vi "HFRR ADV v02.vi"() -> ()   [LabVIEW 2025] (continued)
            frame 9 {
            }
            frame 10 {
              n1911 = local write "Language Selection"(w2311) -> ()
            }
            frame 11 {
            }
            frame 12 {
            }
            frame 13 {
            }
            frame 14 {
            }
            frame 15 {
            }
            frame 16 {
            }
            frame 17 {
            }
            frame 18 {
            }
            frame 21 {
            }
            frame 22 {
              n1912 = local write "Com Port 3"(w2312) -> ()
            }
            frame 20 {
              n1913 = local write "Camera Port :"(w2313) -> ()
            }
            frame 19 {
              n1914 = local write "C3 :"(w2314) -> ()
            }
            frame 23, Default {
            }
          }
        }
      }
    }
    n1915 = Select(t=u32 2500 ("milliseconds to wait"), s=w2281, f=u32 500 ("milliseconds to wait")) -> (s? t:f=w2279:u32)
    n1916 = Multiply(x=w2284, y=w2279) -> (x*y=w2286:dbl)
    n1917 = call "Elapsed Time2"("Time Target (s)"=w2286, "Auto Reset"=TRUE) -> ("Time has Elapsed"=w2276:bool)  [unwired: 10 in, 7 out]
    n1918 = case shown="True" w2276 {
      frame False {
      }
      frame True {
        n1919 = stacked-sequence {
          frame #0 {
            # "DATA PROCESSING"
            # "115 mV/N"
            n1920 = local read "Sample Temperature 2"() -> (w2318:dbl)
            n1921 = local read "DEMO MODE"() -> (w2315:bool)
            n1922 = local read "RH Numeric:"() -> (→"Humidity ( %RH )":dbl)
            n1923 = local read "FRICVALZ"() -> (w2334:dbl)
            n1924 = local read "Friction"() -> (w2320:dbl)
            n1925 = call <vilib>:"Mean PtByPt.vi"("x"=w2318, "sample length"=100) -> ("mean"=w2317:dbl)  [unwired: 2 in, 1 out]
            "TEMP 2" <- w2317
            "TEMP 3" <- w2317
            n1926 = Subtract(x=w2320, y=w2334) -> (x-y=w2329:dbl)
            "FF 2" <- w2329
            "FF 4" <- w2329
            n1927 = case shown="False" w2315 {
              frame False {
                n1928 = local read "Ambient Temperature"() -> (→"AIR TEMP":dbl)
              }
              frame True {
              }
            }
            n1929 = local read "TEMP"() -> (w2333:dbl)
            n1930 = local write "FF 3"(w2329) -> ()
            n1931 = Compound Arithmetic op=OR("FRICVALZ 4", "FRICVALZ 3", "FRICVALZ 2") -> (w2325:bool)
            n1932 = case shown="True" w2325 {
              tunnel: w2320 -> [_ w2341]
              frame False {
              }
              frame True {
                w2340 = FALSE ("FRICVALZ")
                n1933 = local write "FRICVALZ 3"(w2340) -> ()
                n1934 = local write "FRICVALZ 2"(w2340) -> ()
                n1935 = local write "FRICVALZ 4"(w2340) -> ()
                "FRICVALZ" <- w2341
              }
            }
            n1936 = Not A Number/Path/Refnum?(number/path/refnum=w2333) -> (NaN/Path/Refnum?=w2332:bool)
            n1937 = Not A Number/Path/Refnum?(number/path/refnum=w2329) -> (NaN/Path/Refnum?=w2331:bool)
            n1938 = Divide(x=w2329, y=1.96) -> (x/y=w2326:dbl)
            n1939 = Compound Arithmetic op=OR(w2332, w2331) -> (w2330:bool)
            n1940 = Not A Number/Path/Refnum?(number/path/refnum=w2326) -> (NaN/Path/Refnum?=w2327:bool)
            n1941 = case shown="True" w2330 {
              frame False {
              }
              frame True {
                n1942 = local write "TEMP"(0.0 ("TEMP")) -> ()
                n1943 = local write "FF 2"(0.0 ("FF 2")) -> ()
                n1944 = local write "reinit"(TRUE ("reinit")) -> ()
              }
            }
            n1945 = local write "TEMP"(w2317) -> ()
            n1946 = Select(t=0.0, s=w2327, f=w2326) -> (s? t:f=w2319:dbl)
            "COF 2" <- w2319
            n1947 = local write "COF 3"(w2319) -> ()
          }
        }
      }
    }
    n1948 = Wait (ms)(milliseconds to wait=u32 50) -> ()  [unwired: 1 out]
    n1949 = local read "Quit"() -> (w2270:bool)
    "Rate" <- 2500.0 ("No of Samples")
  }
  n1950 = while {
    tunnel: [w2361] -> _
    tunnel: [w2344] -> w59
    tunnel: w7 -> [_]
    i -> [w2361]
    stop <- w2344 stop-if-true
    # "C:\\LAB-IQ-NXT\\Scar View.exe"
    n1951 = local read "OK Button 16"() -> (w2351:bool)
    n1952 = local read "Main Tab"() -> (w2345:T4)
    n1953 = local read "service 3"() -> (w2346:bool)
    n1954 = local read "OPEN 6"() -> (w2348:bool)
    n1955 = local read "EDIT 2"() -> (w2350:bool)
    n1956 = flat-sequence {
      frame #0 {
        n1957 = stacked-sequence {
          frame #0 {
            n1958 = local read "EDIT"() -> (w2839:bool)
            n1959 = case shown="False" w2839 {
              tunnel: [u8 2 ("Disabled") u8 0 ("Disabled")] -> _
              frame False {
                w2841 = FALSE
                n1960 = local write "Password"("") -> ()
                n1961 = local write "x = y?"(w2841) -> ()
                n1962 = property on="Password" class="Str"("Visible"=w2841) -> ()  [unwired: 2 in, 2 out]
              }
              frame True {
                n1963 = property on="Password" class="Str"("Visible"=TRUE) -> ()  [unwired: 2 in, 2 out]
              }
            }
            "dipl pwd" <- "@143$\n" ("dipl pwd")
          }
          frame #1 {
          }
          frame #2 {
          }
          frame #3 {
          }
          frame #4 {
            n1964 = String To Byte Array(string="Password") -> (unsigned byte array=w2852:u8[])
            n1965 = Search 1D Array(1D array=w2852, element=u8 10) -> (index of element=w2850:i32)  [unwired: 1 in]
            n1966 = Index Array(array=w2852, index=w2850) -> (element=w2851:u8)
            n1967 = Equal?(x=w2851, y=10) -> (x = y?=w2847:bool)
            n1968 = case shown="True" w2847 {
              frame False {
              }
              frame True {
                # "password"
                # "password"
                n1969 = local read "Password"() -> (w2864:string)
                n1970 = String To Byte Array(string=w2864) -> (unsigned byte array=w2867:u8[])
                n1971 = String To Byte Array(string="@143$\n") -> (unsigned byte array=w2854:u8[])
                n1972 = Array Size(array=w2867) -> (size(s)=w2863:i32)
                n1973 = Array Size(array=w2854) -> (size(s)=w2859:i32)
                n1974 = for {
                  N: w2863 -> [_]
                  tunnel: w2867 -> [w2880]
                  tunnel: [w2878] -> w2868 mode=indexing
                  tunnel: w2863 -> [w2875]
                  i -> [w2876]
                  n1975 = Decrement(x=w2875) -> (x-1=w2874:i32)
                  n1976 = Index Array(array=w2880, index=w2876) -> (element=w2879:u8)
                  n1977 = Equal?(x=w2876, y=w2874) -> (x = y?=w2873:bool)
                  n1978 = Number To Decimal String(number=w2879) -> (decimal integer string=w2877:string)  [unwired: 1 in]
                  n1979 = Select(t="", s=w2873, f="\r") -> (s? t:f=w2870:string)
                  n1980 = Concatenate Strings(w2877, w2870) -> (w2878:string)
                }
                n1981 = for {
                  N: w2859 -> [_]
                  tunnel: w2854 -> [w2891]
                  tunnel: [w2889] -> w2857 mode=indexing
                  tunnel: w2859 -> [w2886]
                  i -> [w2887]
                  n1982 = Decrement(x=w2886) -> (x-1=w2885:i32)
                  n1983 = Index Array(array=w2891, index=w2887) -> (element=w2890:u8)
                  n1984 = Equal?(x=w2887, y=w2885) -> (x = y?=w2884:bool)
                  n1985 = Number To Decimal String(number=w2890) -> (decimal integer string=w2888:string)  [unwired: 1 in]
                  n1986 = Select(t="", s=w2884, f="\r") -> (s? t:f=w2881:string)
                  n1987 = Concatenate Strings(w2888, w2881) -> (w2889:string)
                }
                n1988 = local read "file path"() -> (w2853:path)
                n1989 = call <vilib>:"Read Characters From File.vi"("file path (dialog if empty)"=w2853) -> ("character string"=w2866:string)  [unwired: 5 in, 3 out]
                "string" <- w2866
                n1990 = flat-sequence {
                  tunnel: [w2869] -> _
                  frame #0 {
                    w2869 = ""
                    n1991 = local write "Password"(w2869) -> ()
                  }
                }
                n1992 = Concatenate Strings(w2857) -> (w2858:string)
                n1993 = Concatenate Strings(w2866) -> (w2865:string)
                n1994 = Concatenate Strings(w2868) -> (w2861:string)
                n1995 = Equal?(x=w2861, y=w2865) -> (x = y?=w2856:bool)
                n1996 = Equal?(x=w2861, y=w2858) -> (x = y?=w2862:bool)
                n1997 = Or(x=w2856, y=w2862) -> (x .or. y?=→"x = y?":bool)
              }
            }
          }
        }
        n1998 = local read "x = y?"() -> (w2837:bool)
        n1999 = And(x="EDIT", y=w2837) -> (x .and. y?=w2835:bool)
        n2000 = case shown="True" w2835 {
          tunnel: [u8 2 ("Disabled") u8 0 ("Disabled")] -> w2834
          tunnel: [w3041 TRUE ("Visible")] -> w2833
          frame False {
            w3041 = FALSE ("Visible")
            n2001 = local write "EDIT 2"(w3041) -> ()
          }
          frame True {
          }
        }
        n2002 = case shown="True" "SAVE" {
          frame False {
          }
          frame True {
            n2003 = stacked-sequence {
              seq-local: [w2896 _ _] -> [_ w3037 _]
              frame #0 {
                w2892 = 0.0 ("number")
                w2893 = 0.0 ("number")
                (unwired) i16 5 ("precision (6)")
                # "[CH1]    - FF\n[CH2]   - TEMPERATURE\n[CH3]    - Humidity\n[CH4]    - AIR TEMP\n[CH5]\\- Visa Uno\n[CH6] \\- Visa Due\n[CH7]  \\- file path\n[CH8]   - Displacement Gain\n[CHA]   - Stroke Gain\n[CHB]   - Stroke PID Gain\n[CHC]   -Language Selection\n[CHD]   -Power +\n[CHE]   -Power_\n[CHF]   -Heater\n[CHG]   -Humidity Wet\n[CHH]   -Humidity Dry\n[CHI]   -Integral Time"
                n2004 = local read "Language Selection"() -> (w2939:enum16{"English", "Russian"})
                n2005 = Path To String(path="File Path") -> (string=w2955:string)
                n2006 = Number To Fractional String(number=w2892, width (-)=i16 10 ("precision (6)"), precision (6)=i16 5) -> (F-format string=w2946:string)  [unwired: 1 in]
                n2007 = Number To Fractional String(number=w2939, width (-)=i16 10 ("precision (6)"), precision (6)=i16 5) -> (F-format string=w2935:string)  [unwired: 1 in]
                n2008 = Number To Fractional String(number=w2893, width (-)=i16 10 ("precision (6)"), precision (6)=i16 5) -> (F-format string=w2929:string)  [unwired: 1 in]
                n2009 = Number To Fractional String(number=w2893, width (-)=i16 10 ("precision (6)"), precision (6)=i16 5) -> (F-format string=w2926:string)  [unwired: 1 in]
                n2010 = Number To Fractional String(number=w2893, width (-)=i16 10 ("precision (6)"), precision (6)=i16 5) -> (F-format string=w2921:string)  [unwired: 1 in]
                n2011 = Number To Fractional String(number=w2893, width (-)=i16 10 ("precision (6)"), precision (6)=i16 5) -> (F-format string=w2918:string)  [unwired: 1 in]
                n2012 = Number To Fractional String(number=w2893, width (-)=i16 10 ("precision (6)"), precision (6)=i16 5) -> (F-format string=w2913:string)  [unwired: 1 in]
                n2013 = local read "Com Port 1"() -> (w2895:refnum<visa-resource-name>)
                n2014 = local read "Com Port 2"() -> (w2894:refnum<visa-resource-name>)
                n2015 = Concatenate Strings(w2955, "\\" ("string")) -> (w2954:string)
                n2016 = Number To Fractional String(number=w2892, width (-)=i16 10 ("precision (6)"), precision (6)=i16 5) -> (F-format string=w2987:string)  [unwired: 1 in]
                n2017 = Number To Fractional String(number=w2892, width (-)=i16 10 ("precision (6)"), precision (6)=i16 5) -> (F-format string=w2986:string)  [unwired: 1 in]
                n2018 = Number To Fractional String(number=w2892, width (-)=i16 10 ("precision (6)"), precision (6)=i16 5) -> (F-format string=w2980:string)  [unwired: 1 in]
                n2019 = Number To Fractional String(number=w2892, width (-)=i16 10 ("precision (6)"), precision (6)=i16 5) -> (F-format string=w2974:string)  [unwired: 1 in]
                n2020 = Number To Fractional String(number=w2892, width (-)=i16 10 ("precision (6)"), precision (6)=i16 5) -> (F-format string=w2947:string)  [unwired: 1 in]
                n2021 = Concatenate Strings("[CHA]" ("string"), w2946, "- Stroke Gain" ("string"), "\r") -> (w2940:string)
                n2022 = Concatenate Strings("[CHC]" ("string"), w2935, "-Language Selection" ("string"), "\r") -> (w2932:string)
                n2023 = Concatenate Strings("[CHD]" ("string"), w2929, "-Power +" ("string"), "\r") -> (w2911:string)
                n2024 = Concatenate Strings("[CHG]" ("string"), w2918, "-Humidity Wet" ("string"), "\r") -> (w2908:string)
                n2025 = Concatenate Strings("[CHH]" ("string"), w2913, "-Humidity Dry" ("string"), "\r") -> (w2907:string)
                n2026 = Concatenate Strings("[CH1]" ("string"), w2987, " - FF" ("string"), "\r") -> (w2985:string)
                n2027 = Concatenate Strings("[CH2]" ("string"), w2986, " - TEMPERATURE" ("string"), "\r") -> (w2984:string)
                n2028 = Concatenate Strings("[CH3]" ("string"), w2980, " - Humidity" ("string"), "\r") -> (w2977:string)
                n2029 = Concatenate Strings("[CH4]" ("string"), w2974, " - AIR TEMP" ("string"), "\r") -> (w2970:string)
                n2030 = Concatenate Strings("[CH5]" ("string"), w2895, "- Visa Uno" ("string"), "\r") -> (w2963:string)
                n2031 = Concatenate Strings("[CH6]" ("string"), w2894, "- Visa Due" ("string"), "\r") -> (w2958:string)
                n2032 = Concatenate Strings("[CH7]" ("string"), w2954, "- file path" ("string"), "\r") -> (w2957:string)
                n2033 = Concatenate Strings("[CH8]" ("string"), w2947, "- Displacement Gain" ("string"), "\r") -> (w2950:string)
                n2034 = Concatenate Strings("[CHE]" ("string"), w2926, "-Power_" ("string"), "\r") -> (w2910:string)
                n2035 = Concatenate Strings("[CHF]" ("string"), w2921, "-Heater" ("string"), "\r") -> (w2909:string)
                n2036 = Concatenate Strings(w2985, w2984, w2977, w2970, w2963, w2958, w2957, w2950, w2940, w2932, w2911, w2910, w2909, w2908, w2907) -> (w2896:string)
                "gain" <- w2896
              }
              frame #1 {
                w2998 = 0.0 ("number")
                n2037 = local read "Camera Port :"() -> (w3001:string)
                n2038 = local read "C3 :"() -> (w3009:refnum<visa-resource-name>)
                n2039 = local read "Com Port 3"() -> (w3010:refnum<visa-resource-name>)
                n2040 = Concatenate Strings("[CH8]" ("string"), w3001, "- Visa Camera" ("string"), "\r") -> (w3000:string)
                n2041 = Concatenate Strings("[CH7]" ("string"), w3009, "- Visa Humidity" ("string"), "\r") -> (w3005:string)
                n2042 = Number To Fractional String(number=w2998, width (-)=i16 10 ("precision (6)"), precision (6)=i16 5) -> (F-format string=w3025:string)  [unwired: 1 in]
                n2043 = Concatenate Strings("[CHL]" ("string"), w3010, "- Visa humid" ("string"), "\r") -> (w3013:string)
                n2044 = Number To Fractional String(number=w2998, width (-)=i16 10 ("precision (6)"), precision (6)=i16 5) -> (F-format string=w3032:string)  [unwired: 1 in]
                n2045 = Concatenate Strings("[CHK]" ("string"), w3025, "-TEMP INTERCEPT" ("string"), "\r") -> (w3021:string)
                n2046 = Concatenate Strings("[SNO]" ("string"), "" ("string"), "-" ("string"), "\r") -> (w3018:string)
                n2047 = Concatenate Strings("[CHJ]" ("string"), w3032, "-AIR TEMP INTERCEPT" ("string"), "\r") -> (w3022:string)
                n2048 = String To Path(string="C:\\LAB-IQ\\calibrate WO 2472.dcf") -> (path=w3011:path)
                n2049 = Concatenate Strings(w3037, w3022, w3021, w3018, w3013, w3005, w3000) -> (w3036:string)
                n2050 = call <vilib>:"Write Characters To File.vi"("append to file? (new file:F)"=FALSE, "character string"=w3036, "file path (dialog if empty)"=w3011) -> ()  [unwired: 2 in, 1 out]
              }
              frame #2 {
                n2051 = local write "Lan flag"(0.0 ("Lan flag")) -> ()
                n2052 = local write "conststatus"(0.0 ("rpm value : 2")) -> ()
                n2053 = local write "SAVE"(FALSE ("OK Button 14")) -> ()
              }
            }
          }
        }
        n2054 = property on="EDIT 2" class="Bool (strict)"("Visible"=w2833) -> ()  [unwired: 2 in, 2 out]
        n2055 = property on="SAVE" class="Bool (strict)"("Visible"=w2833) -> ()  [unwired: 2 in, 2 out]
        n2056 = property on="visa due" class="CmbBox"("Disabled"=w2834) -> ()  [unwired: 2 in, 2 out]
        n2057 = property on="File Path" class="Path"("Disabled"=w2834) -> ()  [unwired: 2 in, 2 out]
        n2058 = property on="Language Selection" class="Enum (strict)"("Visible"=w2833) -> ()  [unwired: 2 in, 2 out]
        n2059 = property on="SPEED OUT:" class="DigNum (strict)"("Disabled"=w2834) -> ()  [unwired: 2 in, 2 out]
      }
    }
    n2060 = local read "RUN"() -> (w2360:bool)
    n2061 = local read "RUN"() -> (w2358:bool)
    n2062 = case shown="True" "EDIT 3" {
      frame False {
      }
      frame True {
        n2063 = local write "EDIT 3"(FALSE ("EDIT 3")) -> ()
        n2064 = local write "Main Tab"(T4."About" ("Main Tab")) -> ()
      }
    }
    n2065 = case shown="False" w2360 {
      frame False {
        n2066 = local read "stopT"() -> (w3048:bool)
        n2067 = case shown="True" w3048 {
          frame False {
          }
          frame True {
            n2068 = local write "stopT"(FALSE) -> ()
          }
        }
      }
      frame True {
        "stopT" <- TRUE
      }
    }
    n2069 = case shown="False" w2358 {
      frame False {
      }
      frame True {
      }
    }
    n2070 = case shown="True" w2350 {
      frame False {
        n2071 = property on="Password 2" class="Str"("Visible"=FALSE) -> ()  [unwired: 2 in, 2 out]
        n2072 = local write "Password 2"("" ("Password")) -> ()
      }
      frame True {
        n2073 = property on="Password 2" class="Str"("Visible"=TRUE) -> ()  [unwired: 2 in, 2 out]
        n2074 = Equal?(x="Password 2", y="HFRR1234") -> (x = y?=w2373:bool)
        n2075 = case shown="True" w2373 {
          tunnel: "Password 2" -> [w2376 _]
          frame False {
            n2076 = String Length(string=w2376) -> (length=w2377:i32)
            n2077 = Greater Than 0?(x=w2377) -> (x > 0?=w2375:bool)
            n2078 = case shown="False" w2375 {
              frame False {
                n2079 = property on="Password 2" class="Str"("Caption.Text"="Password (Advance Setting)") -> ()  [unwired: 2 in, 2 out]
              }
              frame True {
                n2080 = property on="Password 2" class="Str"("Caption.Text"="Incorrect Password!") -> ()  [unwired: 2 in, 2 out]
              }
            }
          }
          frame True {
            n2081 = local write "EDIT 2"(FALSE ("EDIT 2")) -> ()
            n2082 = local write "Password 2"("" ("Password")) -> ()
            n2083 = local write "Main Tab"(T4."Advance" ("Main Tab")) -> ()
            n2084 = local write "Main Dashboard Buttons"(T1."Advance" ("Main Dashboard Buttons")) -> ()
          }
        }
      }
    }
    n2085 = case shown="True" "Prog Uno" {
      frame False {
      }
      frame True {
        n2086 = stacked-sequence {
          frame #0 {
            n2087 = Delete(path (use dialog)=path "C:/LAB-IQ-NXT/UNOCOMPILE.bat" ("working directory")) -> ()  [unwired: 4 in, 3 out]
          }
          frame #1 {
            n2088 = local read "Com Port 1"() -> (w2815:refnum<visa-resource-name>)
            n2089 = Concatenate Strings("cmd.exe /c \"mode " ("command line"), w2815, ":1200,n,8,1\"\n" ("command line")) -> (w2820:string)
            n2090 = Concatenate Strings(w2820, "CD\\\nCD WinDucom\navrdude -C avrdude.conf -v -patmega328p -carduino -P" ("command line"), w2815, " -b115200 -D -Uflash:w:UNO_V20.hex:i\n" ("command line"), "\r") -> (w2822:string)
            "STR" <- w2822
            n2091 = call <vilib>:"Write Characters To File.vi"("append to file? (new file:F)"=FALSE, "character string"=w2822, "file path (dialog if empty)"=path "C:/LAB-IQ/UNOCOMPILE.bat" ("working directory")) -> ()  [unwired: 2 in, 1 out]
          }
          frame #2 {
            n2092 = disable-structure shown="Disabled" {
              frame Disabled {
                w2826 = "cmd.exe  /c \"C:\\LAB-IQ-NXT\\UNOCOMPILE.bat\"" ("string")
                n2093 = local write "Prog Uno"(FALSE ("run minimized? (F)")) -> ()
                n2094 = call <vilib>:"System Exec.vi"("expected output size  (4096)"=u32 65535, "run minimized? (F)"=FALSE, "wait until completion? (T)"=TRUE ("run minimized? (F)"), "working directory"=path "C:/LAB-IQ-NXT", "standard input"=w2826, "command line"=w2826) -> ("error out"=w2825:errorcluster, "standard output"=→"String 42":string)  [unwired: 2 in, 2 out]
                "error out 3" <- w2825
                n2095 = flat-sequence {
                  tunnel: w2825 -> [_]
                  frame #0 {
                  }
                }
              }
              frame Enabled {
              }
            }
          }
        }
      }
    }
    n2096 = case shown="\"ISO 12156\"" "TEST STANDARD" {
      frame "ASTM D6079", Default {
        w2795 = 50.0 ("Hz")
        w2796 = 53.0 ("Set Rh")
        w2798 = 1.0 ("Set Strk")
        w2797 = 60.0 ("Set Temp")
        # "astm hide"
        n2097 = local write "NORMAL LOAD"(200.0 ("NORMAL LOAD")) -> ()
        n2098 = local write "Set Strk"(w2798) -> ()
        n2099 = local write "Set Hz"(w2795) -> ()
        n2100 = local write "Set Temp"(w2797) -> ()
        n2101 = local write "Set Rh"(w2796) -> ()
        n2102 = local write "test time"(75.0 ("test time")) -> ()
        n2103 = local write "Set Stroke:"(w2798) -> ()
        n2104 = local write "Set Humidity:"(w2796) -> ()
        n2105 = local write "Set Frequency:"(w2795) -> ()
        n2106 = local write "Set Temperature:"(w2797) -> ()
        "Test Standard" <- "ASTM D6079" ("Test Standard 2")
      }
      frame "ISO 12156" {
        n2107 = local write "Set Strk"(1.0 ("Set Strk")) -> ()
        n2108 = local write "NORMAL LOAD"(200.0 ("NORMAL LOAD")) -> ()
        n2109 = local write "Set Temp"(60.0 ("Set Temp")) -> ()
        n2110 = local write "test time"(75.0 ("test time")) -> ()
        n2111 = local write "Set Hz"(50.0 ("Hz")) -> ()
        n2112 = local write "Set Rh"(53.0 ("Set Rh")) -> ()
      }
      frame "ASTM D7688" {
        n2113 = local write "Set Strk"(1.0 ("Set Strk")) -> ()
        n2114 = local write "NORMAL LOAD"(200.0 ("NORMAL LOAD")) -> ()
        n2115 = local write "Set Temp"(60.0 ("Set Temp")) -> ()
        n2116 = local write "test time"(75.0 ("test time")) -> ()
        n2117 = local write "Set Hz"(50.0 ("Hz")) -> ()
        n2118 = local write "Set Rh"(53.0 ("Set Rh")) -> ()
      }
      frame "Custom" {
      }
    }
    n2119 = Or(x=w2348, y=w2346) -> (x .or. y?=w2347:bool)
    n2120 = case shown="\"About\"" w2345 {
      tunnel: [T29."Acquire" ("Main Tab") T29."Compare Files" ("Main Tab") T29."About" ("Main Tab")] -> w2356
      frame "Acquire", Default {
      }
      frame "Compare Files" {
      }
      frame "About" {
      }
    }
    n2121 = Or(x=w2351, y="OPEN") -> (x .or. y?=w2352:bool)
    n2122 = case shown="True" w2352 {
      tunnel: w2351 -> [_ w2384]
      frame False {
      }
      frame True {
        n2123 = stacked-sequence {
          tunnel: w2384 -> [_ w2451 _ _]
          frame #0 {
            w2400 = "  " ("String 6")
            n2124 = local write "OPEN"(FALSE ("open")) -> ()
            n2125 = local read "string1 2"() -> (w2388:string)
            n2126 = local read "string1 3"() -> (w2387:string)
            n2127 = local read "string1 4"() -> (w2386:string)
            n2128 = property on="OPEN" class="Bool (strict)"("Visible"=FALSE) -> ()  [unwired: 2 in, 2 out]
            n2129 = local write "String 6"(w2400) -> ()
            n2130 = local write "String 7"(w2400) -> ()
            n2131 = local write "String 8"(w2400) -> ()
            n2132 = local write "String 12"(w2400) -> ()
            n2133 = local read "OK Button 16"() -> (w2385:bool)
            n2134 = String To Path(string=w2388) -> (path=w2396:path)
            n2135 = String To Path(string=w2387) -> (path=w2395:path)
            n2136 = String To Path(string=w2386) -> (path=w2394:path)
            n2137 = case shown="True" w2385 {
              tunnel: [w2401 w2402] -> w2389
              frame False {
                n2138 = local read "string1"() -> (w2401:string)
              }
              frame True {
                n2139 = local read "String Indicator 4"() -> (w2402:string)
              }
            }
            n2140 = Open/Create/Replace File "Open File"(file path (use dialog)=w2396) -> (refnum out=w2392:refnum<file>)  [unwired: 5 in, 2 out]
            n2141 = Open/Create/Replace File "Open File"(file path (use dialog)=w2395) -> (refnum out=w2391:refnum<file>)  [unwired: 5 in, 2 out]
            n2142 = Open/Create/Replace File "Open File"(file path (use dialog)=w2394) -> (refnum out=w2390:refnum<file>)  [unwired: 5 in, 2 out]
            n2143 = while {
              tunnel: w2392 -> [w2414]
              i -> [w2410]
              stop <- w2409 continue-if-true
              (unwired) TRUE ("line mode (F)")
              n2144 = Read from Text File "Read File"(file (use dialog)=w2414) -> (text=w2411:string)  [unwired: 3 in, 3 out]
              n2145 = local write "Numeric 11"(w2410) -> ()
              n2146 = String Length(string=w2411) -> (length=w2413:i32)
              n2147 = Greater?(x=w2413, y=1) -> (0:w2409:bool)
            }
            n2148 = while {
              tunnel: w2391 -> [w2420]
              i -> [w2416]
              stop <- w2415 continue-if-true
              (unwired) TRUE ("line mode (F)")
              n2149 = Read from Text File "Read File"(file (use dialog)=w2420) -> (text=w2417:string)  [unwired: 3 in, 3 out]
              n2150 = local write "Numeric 12"(w2416) -> ()
              n2151 = String Length(string=w2417) -> (length=w2419:i32)
              n2152 = Greater?(x=w2419, y=1) -> (0:w2415:bool)
            }
            n2153 = while {
              tunnel: w2390 -> [w2426]
              i -> [w2422]
              stop <- w2421 continue-if-true
              (unwired) TRUE ("line mode (F)")
              n2154 = Read from Text File "Read File"(file (use dialog)=w2426) -> (text=w2423:string)  [unwired: 3 in, 3 out]
              n2155 = local write "Numeric 13"(w2422) -> ()
              n2156 = String Length(string=w2423) -> (length=w2425:i32)
              n2157 = Greater?(x=w2425, y=1) -> (0:w2421:bool)
            }
            n2158 = String To Path(string=w2389) -> (path=w2397:path)
            n2159 = Open/Create/Replace File "Open File"(file path (use dialog)=w2397) -> (refnum out=w2393:refnum<file>)  [unwired: 5 in, 2 out]
            n2160 = while {
              tunnel: w2393 -> [w2408]
              i -> [w2404]
              stop <- w2403 continue-if-true
              (unwired) TRUE ("line mode (F)")
              n2161 = Read from Text File "Read File"(file (use dialog)=w2408) -> (text=w2405:string)  [unwired: 3 in, 3 out]
              n2162 = local write "Numeric 8"(w2404) -> ()
              n2163 = String Length(string=w2405) -> (length=w2407:i32)
              n2164 = Greater?(x=w2407, y=1) -> (0:w2403:bool)
            }
          }
          frame #1 {
            w2578 = FALSE ("ACTUAL   MERGE")
            # "Sample Temp"
            # "ECR"
            # "COF"
            # "Time\nCOF\nFF\nTemp"
            n2165 = case shown="True" w2451 {
              tunnel: [w2598 w2599] -> w2452
              frame False {
                n2166 = local read "string1"() -> (w2598:string)
              }
              frame True {
                n2167 = local read "String Indicator 4"() -> (w2599:string)
              }
            }
            n2168 = local read "string1 3"() -> (w2496:string)
            n2169 = String To Path(string=w2452) -> (path=w2583:path)
            n2170 = String To Path(string=w2496) -> (path=w2594:path)
            n2171 = local read "Numeric 12"() -> (w2580:i32)
            n2172 = local read "Numeric 8"() -> (w2582:i32)
            n2173 = local read "string1 2"() -> (w2497:string)
            n2174 = local read "string1 4"() -> (w2495:string)
            n2175 = Open/Create/Replace File "Open File"(file path (use dialog)=w2583) -> (refnum out=w2597:refnum<file>, error out=w2596:errorcluster)  [unwired: 5 in, 1 out]
            n2176 = Open/Create/Replace File "Open File"(file path (use dialog)=w2594) -> (refnum out=w2590:refnum<file>, error out=w2591:errorcluster)  [unwired: 5 in, 1 out]
            n2177 = for {
              N: w2582 -> [_]
              tunnel: w2597 -> [w2745]
              tunnel: w2596 -> [w2744]
              tunnel: [w2734] -> w2509 mode=indexing
              tunnel: [w2732] -> w2566 mode=indexing
              tunnel: [w2733] -> w2561 mode=indexing
              tunnel: w2578 -> [_]
              tunnel: [w2726] -> w2563 mode=indexing
              tunnel: [w2722] -> w2532 mode=indexing
              tunnel: [w2718] -> w2507 mode=indexing
              tunnel: [w2714] -> w2488 mode=indexing
              tunnel: [w2709] -> w2448 mode=indexing
              (unwired) TRUE ("line mode (F)")
              # "freq"
              # "Stroke"
              # "Time"
              # "CoF"
              # "Humidity"
              # "Temp"
              # "Air Temp"
              # "ECR"
              n2178 = Read from Text File "Read File"(file (use dialog)=w2745, error in=w2744) -> (text=w2710:string)  [unwired: 2 in, 3 out]
              n2179 = local write "String 6"(w2710) -> ()
              n2180 = String Subset(string=w2710, offset (0)=0, length (rest)=14 ("length (rest)")) -> (substring=w2738:string)
              n2181 = String Subset(string=w2710, offset (0)=35, length (rest)=9 ("length (rest)")) -> (substring=w2735:string)
              n2182 = String Subset(string=w2710, offset (0)=15, length (rest)=9 ("length (rest)")) -> (substring=w2741:string)
              n2183 = Fract/Exp String To Number(string=w2738) -> (number=w2734:dbl)  [unwired: 3 in, 1 out]
              n2184 = Fract/Exp String To Number(string=w2735) -> (number=w2733:dbl)  [unwired: 3 in, 1 out]
              n2185 = Fract/Exp String To Number(string=w2741) -> (number=w2732:dbl)  [unwired: 3 in, 1 out]
              n2186 = String Subset(string=w2710, offset (0)=85, length (rest)=9 ("length (rest)")) -> (substring=w2711:string)
              n2187 = String Subset(string=w2710, offset (0)=25, length (rest)=9 ("length (rest)")) -> (substring=w2717:string)
              n2188 = String Subset(string=w2710, offset (0)=55, length (rest)=9 ("length (rest)")) -> (substring=w2719:string)
              n2189 = String Subset(string=w2710, offset (0)=45, length (rest)=9 ("length (rest)")) -> (substring=w2725:string)
              n2190 = String Subset(string=w2710, offset (0)=65, length (rest)=9 ("length (rest)")) -> (substring=w2731:string)
              n2191 = Fract/Exp String To Number(string=w2717) -> (number=w2714:dbl)  [unwired: 3 in, 1 out]
              n2192 = Fract/Exp String To Number(string=w2711) -> (number=w2709:dbl)  [unwired: 3 in, 1 out]
              n2193 = Fract/Exp String To Number(string=w2719) -> (number=w2718:dbl)  [unwired: 3 in, 1 out]
              n2194 = Fract/Exp String To Number(string=w2725) -> (number=w2722:dbl)  [unwired: 3 in, 1 out]
              n2195 = Fract/Exp String To Number(string=w2731) -> (number=w2728:dbl)  [unwired: 3 in, 1 out]
              n2196 = Add(x=w2728, y=0.0) -> (x+y=w2726:dbl)
            }
            n2197 = for {
              N: w2580 -> [_]
              tunnel: w2591 -> [w2671]
              tunnel: w2590 -> [w2670]
              tunnel: [w2660] -> w2549 mode=indexing
              tunnel: [w2658] -> w2547 mode=indexing
              tunnel: [w2659] -> w2543 mode=indexing
              tunnel: w2578 -> [_]
              tunnel: [w2652] -> w2545 mode=indexing
              tunnel: [w2648] -> w2527 mode=indexing
              tunnel: [w2644] -> w2503 mode=indexing
              tunnel: [w2641] -> w2484 mode=indexing
              tunnel: [w2637] -> w2443 mode=indexing
              (unwired) 9 ("length (rest)")
              (unwired) 9 ("length (rest)")
              (unwired) TRUE ("line mode (F)")
              n2198 = Read from Text File "Read File"(file (use dialog)=w2670, error in=w2671) -> (text=w2638:string)  [unwired: 2 in, 3 out]
              n2199 = local write "String 8"(w2638) -> ()
              n2200 = String Subset(string=w2638, offset (0)=85) -> (substring=w2640:string)  [unwired: 1 in]
              n2201 = String Subset(string=w2638, offset (0)=35, length (rest)=9 ("length (rest)")) -> (substring=w2661:string)
              n2202 = String Subset(string=w2638, offset (0)=55, length (rest)=9 ("length (rest)")) -> (substring=w2646:string)
              n2203 = String Subset(string=w2638, offset (0)=25) -> (substring=w2642:string)  [unwired: 1 in]
              n2204 = String Subset(string=w2638, offset (0)=15, length (rest)=9 ("length (rest)")) -> (substring=w2667:string)
              n2205 = String Subset(string=w2638, offset (0)=0, length (rest)=14 ("length (rest)")) -> (substring=w2664:string)
              n2206 = String Subset(string=w2638, offset (0)=45, length (rest)=9 ("length (rest)")) -> (substring=w2651:string)
              n2207 = String Subset(string=w2638, offset (0)=65, length (rest)=9 ("length (rest)")) -> (substring=w2657:string)
              n2208 = Fract/Exp String To Number(string=w2640) -> (number=w2637:dbl)  [unwired: 3 in, 1 out]
              n2209 = Fract/Exp String To Number(string=w2661) -> (number=w2659:dbl)  [unwired: 3 in, 1 out]
              n2210 = Fract/Exp String To Number(string=w2646) -> (number=w2644:dbl)  [unwired: 3 in, 1 out]
              n2211 = Fract/Exp String To Number(string=w2642) -> (number=w2641:dbl)  [unwired: 3 in, 1 out]
              n2212 = Fract/Exp String To Number(string=w2667) -> (number=w2658:dbl)  [unwired: 3 in, 1 out]
              n2213 = Fract/Exp String To Number(string=w2664) -> (number=w2660:dbl)  [unwired: 3 in, 1 out]
              n2214 = Fract/Exp String To Number(string=w2651) -> (number=w2648:dbl)  [unwired: 3 in, 1 out]
              n2215 = Fract/Exp String To Number(string=w2657) -> (number=w2654:dbl)  [unwired: 3 in, 1 out]
              n2216 = Add(x=w2654, y=0.0) -> (x+y=w2652:dbl)
            }
            n2217 = String To Path(string=w2497) -> (path=w2595:path)
            n2218 = String To Path(string=w2495) -> (path=w2589:path)
            n2219 = local read "Numeric 11"() -> (w2579:i32)
            n2220 = local read "Numeric 13"() -> (w2581:i32)
            n2221 = Open/Create/Replace File "Open File"(file path (use dialog)=w2595) -> (refnum out=w2593:refnum<file>, error out=w2592:errorcluster)  [unwired: 5 in, 1 out]
            n2222 = Open/Create/Replace File "Open File"(file path (use dialog)=w2589) -> (refnum out=w2588:refnum<file>, error out=w2587:errorcluster)  [unwired: 5 in, 1 out]
            n2223 = for {
              N: w2579 -> [_]
              tunnel: w2593 -> [w2708]
              tunnel: w2592 -> [w2707]
              tunnel: [w2697] -> w2559 mode=indexing
              tunnel: [w2695] -> w2557 mode=indexing
              tunnel: [w2696] -> w2552 mode=indexing
              tunnel: w2578 -> [_]
              tunnel: [w2689] -> w2554 mode=indexing
              tunnel: [w2685] -> w2530 mode=indexing
              tunnel: [w2681] -> w2505 mode=indexing
              tunnel: [w2677] -> w2486 mode=indexing
              tunnel: [w2672] -> w2444 mode=indexing
              (unwired) TRUE ("line mode (F)")
              n2224 = Read from Text File "Read File"(file (use dialog)=w2708, error in=w2707) -> (text=w2673:string)  [unwired: 2 in, 3 out]
              n2225 = local write "String 7"(w2673) -> ()
              n2226 = String Subset(string=w2673, offset (0)=85, length (rest)=9 ("length (rest)")) -> (substring=w2676:string)
              n2227 = String Subset(string=w2673, offset (0)=35, length (rest)=9 ("length (rest)")) -> (substring=w2698:string)
              n2228 = String Subset(string=w2673, offset (0)=55, length (rest)=9 ("length (rest)")) -> (substring=w2684:string)
              n2229 = String Subset(string=w2673, offset (0)=25, length (rest)=9 ("length (rest)")) -> (substring=w2678:string)
              n2230 = String Subset(string=w2673, offset (0)=45, length (rest)=9 ("length (rest)")) -> (substring=w2686:string)
              n2231 = String Subset(string=w2673, offset (0)=0, length (rest)=14 ("length (rest)")) -> (substring=w2701:string)
              n2232 = String Subset(string=w2673, offset (0)=15, length (rest)=9 ("length (rest)")) -> (substring=w2704:string)
              n2233 = String Subset(string=w2673, offset (0)=65, length (rest)=9 ("length (rest)")) -> (substring=w2690:string)
              n2234 = Fract/Exp String To Number(string=w2676) -> (number=w2672:dbl)  [unwired: 3 in, 1 out]
              n2235 = Fract/Exp String To Number(string=w2698) -> (number=w2696:dbl)  [unwired: 3 in, 1 out]
              n2236 = Fract/Exp String To Number(string=w2684) -> (number=w2681:dbl)  [unwired: 3 in, 1 out]
              n2237 = Fract/Exp String To Number(string=w2678) -> (number=w2677:dbl)  [unwired: 3 in, 1 out]
              n2238 = Fract/Exp String To Number(string=w2686) -> (number=w2685:dbl)  [unwired: 3 in, 1 out]
              n2239 = Fract/Exp String To Number(string=w2701) -> (number=w2697:dbl)  [unwired: 3 in, 1 out]
              n2240 = Fract/Exp String To Number(string=w2704) -> (number=w2695:dbl)  [unwired: 3 in, 1 out]
              n2241 = Fract/Exp String To Number(string=w2690) -> (number=w2693:dbl)  [unwired: 3 in, 1 out]
              n2242 = Add(x=w2693, y=0.0) -> (x+y=w2689:dbl)
            }
            n2243 = for {
              N: w2581 -> [_]
              tunnel: w2588 -> [w2636]
              tunnel: w2587 -> [w2635]
              tunnel: [w2625] -> w2541 mode=indexing
              tunnel: [w2624] -> w2534 mode=indexing
              tunnel: w2578 -> [_]
              tunnel: [w2613] -> w2539 mode=indexing
              tunnel: [w2618] -> w2536 mode=indexing
              tunnel: [w2614] -> w2526 mode=indexing
              tunnel: [w2609] -> w2501 mode=indexing
              tunnel: [w2605] -> w2482 mode=indexing
              tunnel: [w2600] -> w2442 mode=indexing
              (unwired) 1.0 ("x")
              (unwired) TRUE ("line mode (F)")
              n2244 = Read from Text File "Read File"(file (use dialog)=w2636, error in=w2635) -> (text=w2601:string)  [unwired: 2 in, 3 out]
              n2245 = local write "String 12"(w2601) -> ()
              n2246 = String Subset(string=w2601, offset (0)=85, length (rest)=9 ("length (rest)")) -> (substring=w2603:string)
              n2247 = String Subset(string=w2601, offset (0)=35, length (rest)=9 ("length (rest)")) -> (substring=w2626:string)
              n2248 = String Subset(string=w2601, offset (0)=55, length (rest)=9 ("length (rest)")) -> (substring=w2611:string)
              n2249 = String Subset(string=w2601, offset (0)=25, length (rest)=9 ("length (rest)")) -> (substring=w2607:string)
              n2250 = String Subset(string=w2601, offset (0)=45, length (rest)=9 ("length (rest)")) -> (substring=w2616:string)
              n2251 = String Subset(string=w2601, offset (0)=15, length (rest)=9 ("length (rest)")) -> (substring=w2632:string)
              n2252 = String Subset(string=w2601, offset (0)=0, length (rest)=14 ("length (rest)")) -> (substring=w2629:string)
              n2253 = String Subset(string=w2601, offset (0)=65, length (rest)=9 ("length (rest)")) -> (substring=w2619:string)
              n2254 = Fract/Exp String To Number(string=w2603) -> (number=w2600:dbl)  [unwired: 3 in, 1 out]
              n2255 = Fract/Exp String To Number(string=w2626) -> (number=w2624:dbl)  [unwired: 3 in, 1 out]
              n2256 = Fract/Exp String To Number(string=w2611) -> (number=w2609:dbl)  [unwired: 3 in, 1 out]
              n2257 = Fract/Exp String To Number(string=w2607) -> (number=w2605:dbl)  [unwired: 3 in, 1 out]
              n2258 = Fract/Exp String To Number(string=w2616) -> (number=w2614:dbl)  [unwired: 3 in, 1 out]
              n2259 = Fract/Exp String To Number(string=w2632) -> (number=w2613:dbl)  [unwired: 3 in, 1 out]
              n2260 = Fract/Exp String To Number(string=w2629) -> (number=w2625:dbl)  [unwired: 3 in, 1 out]
              n2261 = Fract/Exp String To Number(string=w2619) -> (number=w2622:dbl)  [unwired: 3 in, 1 out]
              n2262 = Add(x=w2622, y=0.0) -> (x+y=w2618:dbl)
            }
            n2263 = Delete From Array(array=w2484, index=0) -> (array with subset deleted=w2457:dbl[])  [unwired: 1 in, 1 out]
            n2264 = Delete From Array(array=w2547, index=0) -> (array with subset deleted=w2520:dbl[])  [unwired: 1 in, 1 out]
            n2265 = Delete From Array(array=w2527, index=0) -> (array with subset deleted=w2515:dbl[])  [unwired: 1 in, 1 out]
            n2266 = Delete From Array(array=w2545, index=0) -> (array with subset deleted=w2546:dbl[])  [unwired: 1 in, 1 out]
            n2267 = call-poly <vilib>:"Mean.vi"("X"=w2457) -> ("mean"=→"КОФ2 4":dbl)  [unwired: 1 out]
            n2268 = call-poly <vilib>:"Mean.vi"("X"=w2520) -> ("mean"=→"КОФ3":dbl)  [unwired: 1 out]
            n2269 = call-poly <vilib>:"Mean.vi"("X"=w2515) -> ("mean"=→"CP3":dbl)  [unwired: 1 out]
            n2270 = Delete From Array(array=w2509, index=0) -> (array with subset deleted=w2436:dbl[])  [unwired: 1 in, 1 out]
            n2271 = Delete From Array(array=w2448, index=0) -> (array with subset deleted=w2435:dbl[])  [unwired: 1 in, 1 out]
            n2272 = Delete From Array(array=w2488, index=0) -> (array with subset deleted=w2459:dbl[])  [unwired: 1 in, 1 out]
            n2273 = Delete From Array(array=w2566, index=0) -> (array with subset deleted=w2521:dbl[])  [unwired: 1 in, 1 out]
            n2274 = Delete From Array(array=w2532, index=0) -> (array with subset deleted=w2517:dbl[])  [unwired: 1 in, 1 out]
            "array w/ subset deleted" <- w2517
            n2275 = Delete From Array(array=w2563, index=0) -> (array with subset deleted=w2564:dbl[])  [unwired: 1 in, 1 out]
            n2276 = call-poly <vilib>:"Mean.vi"("X"=w2459) -> ("mean"=→"КОФ2 2":dbl)  [unwired: 1 out]
            n2277 = call-poly <vilib>:"Mean.vi"("X"=w2521) -> ("mean"=→"КОФ1":dbl)  [unwired: 1 out]
            n2278 = Bundle "Bundle"(w2436, w2435) -> (w2441:cluster{dbl[], dbl[]})  [unwired: 1 in]
            n2279 = Bundle "Bundle"(w2436, w2564) -> (w2428:cluster{dbl[], dbl[]})  [unwired: 1 in]
            n2280 = Delete From Array(array=w2443, index=0) -> (array with subset deleted=w2431:dbl[])  [unwired: 1 in, 1 out]
            n2281 = Delete From Array(array=w2444, index=0) -> (array with subset deleted=w2433:dbl[])  [unwired: 1 in, 1 out]
            n2282 = Delete From Array(array=w2554, index=0) -> (array with subset deleted=w2555:dbl[])  [unwired: 1 in, 1 out]
            n2283 = Delete From Array(array=w2442, index=0) -> (array with subset deleted=w2429:dbl[])  [unwired: 1 in, 1 out]
            n2284 = Delete From Array(array=w2536, index=0) -> (array with subset deleted=w2537:dbl[])  [unwired: 1 in, 1 out]
            n2285 = Delete From Array(array=w2561, index=0) -> (array with subset deleted=w2467:dbl[])  [unwired: 1 in, 1 out]
            n2286 = Delete From Array(array=w2507, index=0) -> (array with subset deleted=w2463:dbl[])  [unwired: 1 in, 1 out]
            n2287 = Delete From Array(array=w2543, index=0) -> (array with subset deleted=w2465:dbl[])  [unwired: 1 in, 1 out]
            n2288 = Delete From Array(array=w2503, index=0) -> (array with subset deleted=w2461:dbl[])  [unwired: 1 in, 1 out]
            n2289 = Delete From Array(array=w2552, index=0) -> (array with subset deleted=w2466:dbl[])  [unwired: 1 in, 1 out]
            n2290 = Delete From Array(array=w2505, index=0) -> (array with subset deleted=w2462:dbl[])  [unwired: 1 in, 1 out]
            n2291 = Delete From Array(array=w2486, index=0) -> (array with subset deleted=w2458:dbl[])  [unwired: 1 in, 1 out]
            n2292 = Delete From Array(array=w2530, index=0) -> (array with subset deleted=w2516:dbl[])  [unwired: 1 in, 1 out]
            n2293 = Delete From Array(array=w2557, index=0) -> (array with subset deleted=w2518:dbl[])  [unwired: 1 in, 1 out]
            n2294 = Delete From Array(array=w2534, index=0) -> (array with subset deleted=w2464:dbl[])  [unwired: 1 in, 1 out]
            n2295 = Delete From Array(array=w2501, index=0) -> (array with subset deleted=w2460:dbl[])  [unwired: 1 in, 1 out]
            n2296 = Delete From Array(array=w2482, index=0) -> (array with subset deleted=w2456:dbl[])  [unwired: 1 in, 1 out]
            n2297 = Delete From Array(array=w2526, index=0) -> (array with subset deleted=w2514:dbl[])  [unwired: 1 in, 1 out]
            n2298 = Delete From Array(array=w2539, index=0) -> (array with subset deleted=w2519:dbl[])  [unwired: 1 in, 1 out]
            n2299 = Delete From Array(array=w2549, index=0) -> (array with subset deleted=w2432:dbl[])  [unwired: 1 in, 1 out]
            n2300 = Delete From Array(array=w2559, index=0) -> (array with subset deleted=w2434:dbl[])  [unwired: 1 in, 1 out]
            n2301 = Delete From Array(array=w2541, index=0) -> (array with subset deleted=w2430:dbl[])  [unwired: 1 in, 1 out]
            n2302 = Bundle "Bundle"(w2436, w2467) -> (w2454:cluster{dbl[], dbl[]})  [unwired: 1 in]
            n2303 = Bundle "Bundle"(w2436, w2521) -> (w2455:cluster{dbl[], dbl[]})  [unwired: 1 in]
            n2304 = Bundle "Bundle"(w2467, w2463) -> (w2469:cluster{dbl[], dbl[]})  [unwired: 1 in]
            n2305 = Bundle "Bundle"(w2432, w2431) -> (w2439:cluster{dbl[], dbl[]})  [unwired: 1 in]
            n2306 = Bundle "Bundle"(w2465, w2461) -> (w2471:cluster{dbl[], dbl[]})  [unwired: 1 in]
            n2307 = Bundle "Bundle"(w2432, w2465) -> (w2575:cluster{dbl[], dbl[]})  [unwired: 1 in]
            n2308 = Bundle "Bundle"(w2432, w2461) -> (w2499:cluster{dbl[], dbl[]})  [unwired: 1 in]
            n2309 = Bundle "Bundle"(w2432, w2520) -> (w2585:cluster{dbl[], dbl[]})  [unwired: 1 in]
            n2310 = Bundle "Bundle"(w2432, w2515) -> (w2523:cluster{dbl[], dbl[]})  [unwired: 1 in]
            n2311 = Bundle "Bundle"(w2432, w2546) -> (w2570:cluster{dbl[], dbl[]})  [unwired: 1 in]
            n2312 = Bundle "Bundle"(w2466, w2462) -> (w2470:cluster{dbl[], dbl[]})  [unwired: 1 in]
            n2313 = Bundle "Bundle"(w2434, w2433) -> (w2440:cluster{dbl[], dbl[]})  [unwired: 1 in]
            n2314 = Bundle "Bundle"(w2434, w2466) -> (w2577:cluster{dbl[], dbl[]})  [unwired: 1 in]
            n2315 = Bundle "Bundle"(w2434, w2462) -> (w2500:cluster{dbl[], dbl[]})  [unwired: 1 in]
            n2316 = Bundle "Bundle"(w2434, w2516) -> (w2524:cluster{dbl[], dbl[]})  [unwired: 1 in]
            n2317 = Bundle "Bundle"(w2434, w2518) -> (w2586:cluster{dbl[], dbl[]})  [unwired: 1 in]
            n2318 = Bundle "Bundle"(w2434, w2555) -> (w2568:cluster{dbl[], dbl[]})  [unwired: 1 in]
            n2319 = Bundle "Bundle"(w2464, w2460) -> (w2472:cluster{dbl[], dbl[]})  [unwired: 1 in]
            n2320 = Bundle "Bundle"(w2430, w2429) -> (w2438:cluster{dbl[], dbl[]})  [unwired: 1 in]
            n2321 = Bundle "Bundle"(w2430, w2464) -> (w2576:cluster{dbl[], dbl[]})  [unwired: 1 in]
            n2322 = Bundle "Bundle"(w2430, w2460) -> (w2498:cluster{dbl[], dbl[]})  [unwired: 1 in]
            n2323 = Bundle "Bundle"(w2430, w2514) -> (w2522:cluster{dbl[], dbl[]})  [unwired: 1 in]
            n2324 = Bundle "Bundle"(w2430, w2519) -> (w2584:cluster{dbl[], dbl[]})  [unwired: 1 in]
            n2325 = Bundle "Bundle"(w2430, w2537) -> (w2569:cluster{dbl[], dbl[]})  [unwired: 1 in]
            n2326 = call-poly <vilib>:"Mean.vi"("X"=w2517) -> ("mean"=→"CP1":dbl)  [unwired: 1 out]
            n2327 = call-poly <vilib>:"Mean.vi"("X"=w2458) -> ("mean"=→"КОФ2 3":dbl)  [unwired: 1 out]
            n2328 = call-poly <vilib>:"Mean.vi"("X"=w2516) -> ("mean"=→"CP2":dbl)  [unwired: 1 out]
            n2329 = call-poly <vilib>:"Mean.vi"("X"=w2518) -> ("mean"=→"КОФ2":dbl)  [unwired: 1 out]
            n2330 = call-poly <vilib>:"Mean.vi"("X"=w2456) -> ("mean"=→"КОФ2 5":dbl)  [unwired: 1 out]
            n2331 = call-poly <vilib>:"Mean.vi"("X"=w2514) -> ("mean"=→"CP4":dbl)  [unwired: 1 out]
            n2332 = call-poly <vilib>:"Mean.vi"("X"=w2519) -> ("mean"=→"КОФ4":dbl)  [unwired: 1 out]
            n2333 = Bundle "Bundle"(w2436, w2463) -> (w2427:cluster{dbl[], dbl[]})  [unwired: 1 in]
            n2334 = Bundle "Bundle"(w2436, w2517) -> (w2450:cluster{dbl[], dbl[]})  [unwired: 1 in]
            n2335 = Build Array "Build Array"(w2427, w2450) -> (w2453:cluster{dbl[], dbl[]}[])
            "XY Graph 17" <- w2453
            n2336 = Build Array "Build Array"(w2441, w2440, w2439, w2438) -> (→"Frequency ( Hz )":cluster{dbl[], dbl[]}[])
            n2337 = Build Array "Build Array"(w2469, w2470, w2471, w2472) -> (→"Air Temp ( °C ) vs Humidity ( % RH )":cluster{dbl[], dbl[]}[])
            n2338 = Build Array "Build Array"(w2454, w2577, w2575, w2576) -> (→"Air Temperature  ( °C )":cluster{dbl[], dbl[]}[])
            n2339 = Build Array "Build Array"(w2427, w2500, w2499, w2498) -> (→"Humidity ( %RH )":cluster{dbl[], dbl[]}[])
            n2340 = Build Array "Build Array"(w2455, w2586, w2585, w2584) -> (→"Coefficient Of Friction":cluster{dbl[], dbl[]}[])
            n2341 = Build Array "Build Array"(w2450, w2524, w2523, w2522) -> (→"Sample Temperature ( °C )":cluster{dbl[], dbl[]}[])
            n2342 = Build Array "Build Array"(w2428, w2568, w2570, w2569) -> (→"XY Graph 13":cluster{dbl[], dbl[]}[])
            n2343 = Bundle "Bundle"(w2436, w2459) -> (w2481:cluster{dbl[], dbl[]})  [unwired: 1 in]
            n2344 = Bundle "Bundle"(w2432, w2457) -> (w2479:cluster{dbl[], dbl[]})  [unwired: 1 in]
            n2345 = Bundle "Bundle"(w2434, w2458) -> (w2480:cluster{dbl[], dbl[]})  [unwired: 1 in]
            n2346 = Bundle "Bundle"(w2430, w2456) -> (w2478:cluster{dbl[], dbl[]})  [unwired: 1 in]
            n2347 = Build Array "Build Array"(w2481, w2480, w2479, w2478) -> (→"Stroke ( mm )":cluster{dbl[], dbl[]}[])
            n2348 = local write "XY Graph 16"(w2453) -> ()
          }
          frame #2 {
          }
          frame #3 {
            n2349 = local write "Numeric 8"(0 ("Numeric 8")) -> ()
            n2350 = local write "Numeric 11"(0 ("Numeric 11")) -> ()
            n2351 = local write "Numeric 12"(0 ("Numeric 12")) -> ()
            n2352 = local write "Numeric 13"(0 ("Numeric 13")) -> ()
            n2353 = property on="OPEN" class="Bool (strict)"("Visible"=TRUE) -> ()  [unwired: 2 in, 2 out]
            n2354 = local read "String Control 2"() -> (w2753:string)
            n2355 = local read "String Control 4"() -> (w2752:string)
            n2356 = local read "String Control 6"() -> (w2751:string)
            n2357 = local read "String Control 8"() -> (w2750:string)
            n2358 = Match Pattern(string=w2753, regular expression="Samples / cycle :- ") -> (after substring=w2767:string)  [unwired: 1 in, 3 out]
            n2359 = Match Pattern(string=w2753, regular expression="Frequency :- ") -> (after substring=w2786:string)  [unwired: 1 in, 3 out]
            n2360 = Match Pattern(string=w2752, regular expression="Samples / cycle :- ") -> (after substring=w2763:string)  [unwired: 1 in, 3 out]
            n2361 = Match Pattern(string=w2752, regular expression="Frequency :- ") -> (after substring=w2781:string)  [unwired: 1 in, 3 out]
            n2362 = Match Pattern(string=w2751, regular expression="Samples / cycle :- ") -> (after substring=w2759:string)  [unwired: 1 in, 3 out]
            n2363 = Match Pattern(string=w2751, regular expression="Frequency :- ") -> (after substring=w2776:string)  [unwired: 1 in, 3 out]
            n2364 = Match Pattern(string=w2750, regular expression="Samples / cycle :- ") -> (after substring=w2755:string)  [unwired: 1 in, 3 out]
            n2365 = Match Pattern(string=w2750, regular expression="Frequency :- ") -> (after substring=w2771:string)  [unwired: 1 in, 3 out]
            n2366 = String Subset(string=w2767, length (rest)=6 ("length (rest)")) -> (substring=w2769:string)  [unwired: 1 in]
            n2367 = String Subset(string=w2786, length (rest)=9 ("length (rest)")) -> (substring=w2788:string)  [unwired: 1 in]
            n2368 = String Subset(string=w2763, length (rest)=6 ("length (rest)")) -> (substring=w2765:string)  [unwired: 1 in]
            n2369 = String Subset(string=w2781, length (rest)=9 ("length (rest)")) -> (substring=w2783:string)  [unwired: 1 in]
            n2370 = String Subset(string=w2759, length (rest)=6 ("length (rest)")) -> (substring=w2761:string)  [unwired: 1 in]
            n2371 = String Subset(string=w2776, length (rest)=9 ("length (rest)")) -> (substring=w2778:string)  [unwired: 1 in]
            n2372 = String Subset(string=w2755, length (rest)=6 ("length (rest)")) -> (substring=w2757:string)  [unwired: 1 in]
            n2373 = String Subset(string=w2771, length (rest)=9 ("length (rest)")) -> (substring=w2773:string)  [unwired: 1 in]
            n2374 = Fract/Exp String To Number(string=w2769) -> (number=w2749:dbl)  [unwired: 3 in, 1 out]
            n2375 = Fract/Exp String To Number(string=w2788) -> (number=w2789:dbl)  [unwired: 3 in, 1 out]
            n2376 = Fract/Exp String To Number(string=w2765) -> (number=w2748:dbl)  [unwired: 3 in, 1 out]
            n2377 = Fract/Exp String To Number(string=w2783) -> (number=w2784:dbl)  [unwired: 3 in, 1 out]
            n2378 = Fract/Exp String To Number(string=w2761) -> (number=w2747:dbl)  [unwired: 3 in, 1 out]
            n2379 = Fract/Exp String To Number(string=w2778) -> (number=w2779:dbl)  [unwired: 3 in, 1 out]
            n2380 = Fract/Exp String To Number(string=w2757) -> (number=w2746:dbl)  [unwired: 3 in, 1 out]
            n2381 = Fract/Exp String To Number(string=w2773) -> (number=w2774:dbl)  [unwired: 3 in, 1 out]
            n2382 = local write "sample1"(w2749) -> ()
            n2383 = local write "freq1"(w2789) -> ()
            n2384 = local write "sample2"(w2748) -> ()
            n2385 = local write "freq2"(w2784) -> ()
            n2386 = local write "sample3"(w2747) -> ()
            n2387 = local write "freq3"(w2779) -> ()
            n2388 = local write "sample4"(w2746) -> ()
            n2389 = local write "freq 4"(w2774) -> ()
          }
        }
      }
    }
    n2390 = case shown="True" w2347 {
      selector: w2347 -> [_ w2366]
      frame False {
      }
      frame True {
        n2391 = Not(x=w2366) -> (.not. x?=w2362:bool)
        n2392 = local write "service 3"(w2362) -> ()
        n2393 = local write "OPEN 6"(w2362) -> ()
        n2394 = call <vilib>:"System Exec.vi"("wait until completion? (T)"=TRUE, "command line"="C:\\LAB-IQ\\Scar View.exe") -> ("error out"=→"error out 5":errorcluster)  [unwired: 6 in, 3 out]
      }
    }
    n2395 = case shown="\"Acquire\", Default" w2356 {
      frame "Acquire", Default {
        # "Elapsed time\ncof\nstroke\nAir temp\nTemp\nHumidity"
        n2396 = stacked-sequence {
          frame #0 {
            n2397 = case shown="True" "RST FF" {
              frame False {
              }
              frame True {
                w3110 = 0.0 ("X Scale.Range:Maximum")
                n2398 = property on="Frictional Force ( N )" class="WFChart (strict)"("XScale.Maximum"=600.0 ("X Scale.Range:Maximum"), "XScale.Minimum"=w3110, "YScale.Maximum"=10.0 ("Y Scale.Range:Maximum"), "YScale.Minimum"=w3110) -> ()  [unwired: 2 in, 2 out]
              }
            }
          }
          frame #1 {
            n2399 = case shown="True" "RST TEMP" {
              frame False {
              }
              frame True {
                n2400 = property on="Temperature ( Deg C )" class="WFChart (strict)"("XScale.Minimum"=0.0 ("X Scale.Range:Minimum"), "XScale.Maximum"=600.0 ("X Scale.Range:Maximum"), "YScale.Minimum"=0.0 ("Y Scale.Range:Minimum"), "YScale.Maximum"=100.0 ("Y Scale.Range:Maximum")) -> ()  [unwired: 2 in, 2 out]
              }
            }
          }
          frame #2 {
            n2401 = case shown="True" "RSTCOF" {
              frame False {
              }
              frame True {
                n2402 = property on="Coefficient of Friction" class="WFChart (strict)"("XScale.Minimum"=0.0 ("X Scale.Range:Minimum"), "XScale.Maximum"=600.0 ("X Scale.Range:Maximum"), "YScale.Maximum"=1.0 ("X Scale.Range:Minimum"), "YScale.Minimum"=0.0 ("X Scale.Range:Minimum")) -> ()  [unwired: 2 in, 2 out]
              }
            }
          }
          frame #3 {
            n2403 = case shown="True" "RSTCOF 2" {
              frame False {
              }
              frame True {
                (unwired) 100.0 ("Y Scale.Range:Maximum")
                (unwired) 0.0 ("Y Scale.Range:Minimum")
                (unwired) 600.0 ("X Scale.Range:Maximum")
                (unwired) 0.0 ("X Scale.Range:Minimum")
              }
            }
          }
          frame #4 {
            n2404 = case shown="True" "RSTCOF 3" {
              frame False {
              }
              frame True {
                n2405 = property on="Electrical Contact Resistance ( % ) 2" class="WFChart (strict)"("XScale.Minimum"=0.0 ("X Scale.Range:Minimum"), "XScale.Maximum"=600.0 ("X Scale.Range:Maximum"), "YScale.Minimum"=0.0 ("Y Scale.Range:Minimum"), "YScale.Maximum"=100.0 ("Y Scale.Range:Maximum")) -> ()  [unwired: 2 in, 2 out]
              }
            }
          }
        }
        n2406 = local read "RUN"() -> (w3055:bool)
        n2407 = case shown="False" w3055 {
          frame False {
          }
          frame True {
          }
        }
        n2408 = local read "RUN"() -> (w3059:bool)
        n2409 = case shown="False" w3059 {
          tunnel: [FALSE ("TEST RUNNING") TRUE ("TEST RUNNING")] -> w3058
          frame False {
            w3129 = 0.0 ("Flag")
            n2410 = local write "Elapsed time"(0.0 ("elapsedtime")) -> ()
            n2411 = local write "Time Remaining"(w3129) -> ()
            n2412 = local write "Flag"(w3129) -> ()
            n2413 = local write "Remaining Time"(w3129) -> ()
          }
          frame True {
            n2414 = local write "Flag"(10.0 ("Flag")) -> ()
          }
        }
        n2415 = local read "AIR TEMP"() -> (w3053:dbl)
        n2416 = Greater Or Equal?(x=w3053, y=15.0) -> (x >= y?=w3054:bool)
        "powstat" <- w3054
        n2417 = case shown="True" "Save & Continue" {
          frame False {
          }
          frame True {
            n2418 = local read "USER ID"() -> (w3432:string)
            n2419 = local read "FILE"() -> (w3440:string)
            n2420 = String Length(string=w3440) -> (length=w3438:i32)
            n2421 = String Length(string=w3432) -> (length=w3435:i32)
            n2422 = Greater?(x=w3438, y=0) -> (0:w3437:bool)
            n2423 = Greater?(x=w3435, y=0) -> (0:w3434:bool)
            n2424 = And(x=w3437, y=w3434) -> (x .and. y?=w3433:bool)
            n2425 = case shown="True" w3433 {
              frame False {
                n2426 = stacked-sequence {
                  frame #0 {
                    n2427 = One Button Dialog(message="Please Enter a File Name and Operator ID to save data !", button name ("OK")="Ok") -> ()  [unwired: 1 out]
                  }
                  frame #1 {
                    n2428 = local write "Save & Continue"(FALSE ("OK Button")) -> ()
                  }
                }
                n2429 = local write "Save & Continue"(FALSE ("OK Button")) -> ()
              }
              frame True {
                n2430 = stacked-sequence {
                  frame #0 {
                    n2431 = local read "FILE"() -> (w3446:string)
                    n2432 = call "file check.vi"("file name in"=w3446) -> ("file name out"=w3445:string)  [unwired: 9 in, 1 out]
                    n2433 = call <vilib>:"Application Directory.vi"() -> ("Application Directory"=w3456:path)
                    n2434 = Build Path(base path=w3456, name or relative path="data") -> (appended path=w3455:path)
                    n2435 = call <vilib>:"Trim Whitespace.vi"("string"=w3445) -> ("trimmed string"=w3453:string)  [unwired: 1 in]
                    n2436 = call <vilib>:"Trim Whitespace.vi"("string"=w3445) -> ("trimmed string"=w3454:string)  [unwired: 1 in]
                    n2437 = List Folder(path=w3455) -> (folder names=w3451:string[])  [unwired: 3 in, 3 out]
                    n2438 = Match Pattern(string=w3453, regular expression="_(") -> (before substring=w3450:string)  [unwired: 1 in, 3 out]
                    n2439 = for {
                      tunnel: w3451 -> [w3465] mode=indexing
                      tunnel: w3450 -> [w3463]
                      shift-right: [w3461] -> w3448
                      shift-left: bool[] [] -> [w3462]
                      n2440 = Match Pattern(string=w3465, regular expression="_(") -> (before substring=w3464:string)  [unwired: 1 in, 3 out]
                      n2441 = Equal?(x=w3464, y=w3463) -> (x = y?=w3460:bool)
                      n2442 = case shown="True" w3460 {
                        tunnel: w3460 -> [_ w3468]
                        tunnel: w3462 -> [w3467 w3470]
                        tunnel: [w3467 w3469] -> w3461
                        frame False {
                        }
                        frame True {
                          n2443 = Insert Into Array(array=w3470, new element=w3468) -> (w3469:bool[])  [unwired: 1 in]
                        }
                      }
                    }
                    n2444 = Equal?(x=w3451, y=w3450) -> (x = y?=w3459:bool[])
                    n2445 = Or Array Elements(Boolean array=w3459) -> (logical OR=w3458:bool)
